vi "Pre Launch Init.vi"(11 "H3611i Actor in":refnum<class "H3611i Actor.lvclass">) -> (0 "error out":errorcluster, 3 "H3611i Actor out":refnum<class "H3611i Actor.lvclass">)   [LabVIEW 2018, in "H3611i.lvlib" / "H3611i Actor.lvclass"]
doc: "Sends a high priority message to it's self to notify the monitor that it's spawned. If it's in the runtime environment, this message is never sent, meaning the monitor will never spawn\n\nCopyright: MGI\nAuthored by: Derek Trepanier"
uses:
  H3611i Actor.lvclass
  C:/Program Files (x86)/National Instruments/LabVIEW 2018/vi.lib/ActorFramework/Actor/Actor.lvclass
  C:/Users/dev/Documents/CODE/LabVIEW/microwaveverify/trunk/MWWL Verification/Sensor Actor/Sensor/Sensor.lvclass
  Datalogger Actor/Datalogger Actor.lvclass
  H3611i Actor.lvclass/H3611i Actor.ctl
  Sensor Actor/Sensor/Sensor.lvclass
  <vilib>/ActorFramework/Actor/Actor.lvclass
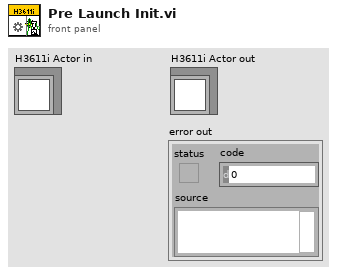
[diagram p1: front panel]
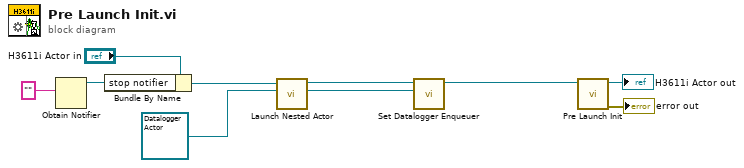
[diagram p0: block diagram]
diagram:
  n1 = Obtain Notifier(notification data type="") -> (notifier out=w6:refnum<notifier>)  [unwired: 3 in, 2 out]
  n2 = Bundle By Name(cluster="H3611i Actor in", "stop notifier"=w6) -> (w4:refnum<class "H3611i Actor.lvclass">)
  n3 = call <vilib>:"Launch Nested Actor.vi"("Nested Actor"=refnum<class "Datalogger Actor.lvclass"> refnum ("Datalogger.lvlib:Datalogger Actor"), "Caller Actor in"=w4) -> ("Nested Actor's Enqueuer"=w2:refnum<class "Message Enqueuer.lvclass">, "Caller Actor out"=w3:refnum<class "H3611i Actor.lvclass">)  [unwired: 7 in, 1 out]
  n4 = call "Set Datalogger Enqueuer.vi"("Datalogger Enqueuer"=w2, "Sensor in"=w3) -> ("Sensor out"=w5:refnum<class "H3611i Actor.lvclass">)  [unwired: 8 in, 1 out]
  n5 = call-parent "Pre Launch Init.vi"("Sensor in"=w5) -> ("error out"=→"error out":errorcluster, "Sensor out"=→"H3611i Actor out":refnum<class "H3611i Actor.lvclass">)  [unwired: 9 in]
